vi "Mixer.Write Mute.vi"(0 "baseURL":string="http://169.254.128.32/datastore/", 7 "mute":bool, 11 "error in (no error)":errorcluster) -> (15 "error out":errorcluster)   [LabVIEW 2020]
uses:
  <vilib>/httpClient/POSTBuffer.vi
  <vilib>/httpClient/LabVIEWHTTPClient.lvlib
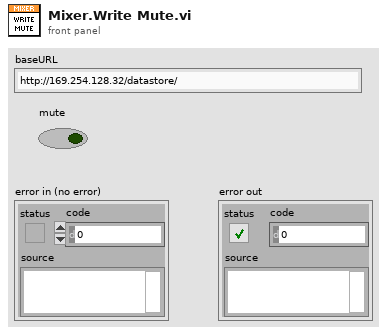
[diagram p1: front panel]
types:
  T1 = typedef "LabVIEWHTTPClient.lvlib/ClientHandle.ctl" = refnum<k1>
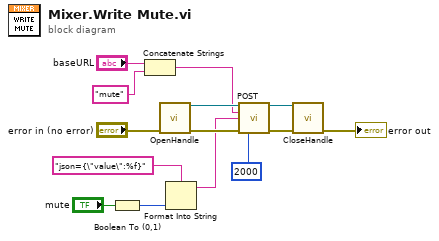
[diagram p0: block diagram]
diagram:
  n1 = Boolean To (0,1)(Boolean="mute") -> (0, 1=w3:i16)
  n2 = Concatenate Strings("baseURL", "mute") -> (w8:string)
  n3 = call <vilib>:"OpenHandle.vi"("error in (no error)"="error in (no error)") -> ("client handle out"=w11:T1, "error out"=w10:errorcluster)  [unwired: 13 in]
  n4 = Format Into String(format string="json={\"value\":%f}" ("buffer"), w3) -> (resulting string=w4:string)  [unwired: 2 in, 1 out]
  n5 = call-poly <vilib>:"POST.vi"("client handle"=w11, "url"=w8, "buffer"=w4, "error in (no error)"=w10, "timeout (10000)"=2000) -> ("client handle out"=w13:T1, "error out"=w14:errorcluster)  [unwired: 7 in, 2 out]
  n6 = call <vilib>:"CloseHandle.vi"("client handle"=w13, "error in (no error)"=w14) -> ("error out"=→"error out":errorcluster)  [unwired: 13 in]
